vi "Test Ping.vi"(8 "error in (no error)":errorcluster) -> (0 "error out":errorcluster, 2 "x = y?":bool)   [LabVIEW 2017]
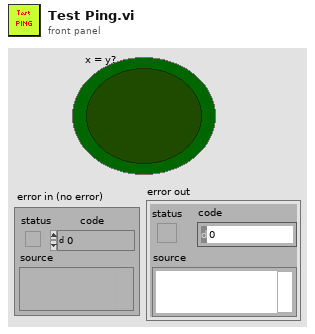
[diagram p1: front panel]
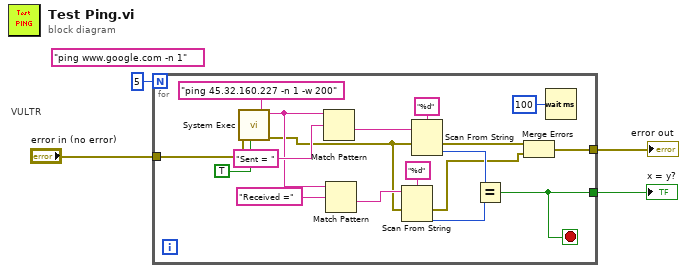
[diagram p0: block diagram]
diagram:
  (unwired) "ping www.google.com -n 1" ("command line")
  # "VULTR"
  n1 = for {
    N: 5 -> [_]
    tunnel: [w6] -> w4
    tunnel: "error in (no error)" -> [w13]
    tunnel: [w9] -> w2
    stop <- w6 stop-if-true
    n2 = call <vilib>:"System Exec.vi"("run minimized? (F)"=TRUE, "error in (no error)"=w13, "command line"="ping 45.32.160.227 -n 1 -w 200") -> ("error out"=w12:errorcluster, "standard output"=w14:string)  [unwired: 5 in, 2 out]
    n3 = Match Pattern(string=w14, regular expression="Sent = ") -> (after substring=w20:string)  [unwired: 1 in, 3 out]
    n4 = Match Pattern(string=w14, regular expression="Received =") -> (after substring=w17:string)  [unwired: 1 in, 3 out]
    n5 = Scan From String(format string="%d", input string=w17, error in=w12) -> (error out=w10:errorcluster, output 1=w15:i32)  [unwired: 2 in, 2 out]
    n6 = Scan From String(format string="%d", input string=w20, error in=w12) -> (error out=w11:errorcluster, output 1=w16:i32)  [unwired: 2 in, 2 out]
    n7 = Equal?(x=w16, y=w15) -> (x = y?=w6:bool)
    n8 = Merge Errors(w11, w10) -> (w9:errorcluster)
    n9 = Wait (ms)(milliseconds to wait=u32 100) -> ()  [unwired: 1 out]
  }
  "x = y?" <- w4
  "error out" <- w2
